vi "ReadByteArray.vi"(0 "Siemens Ctr":T1, 1 "# DB No.":u16, 2 "#items":u16, 3 "Item offset [byte]":u32, 4 "Address Areas":T2=132 items=["Input(I)"=129, "Output(Q)"=130, "Bit Memory(M)"=131, "Data(DB)"=132], 5 "error in (no error)":errorcluster, 6 "Bit/Byte":u8(ring)=2 items=["Boolen"=1, "Byte"=2]) -> (14 "Siemens Ctr out":T1, 15 "Byte Array":u8[](array[numeric]), 19 "error out":errorcluster)   [LabVIEW 2014, in "Simatic S7.lvlib"]
uses:
  Simatic S7.lvlib
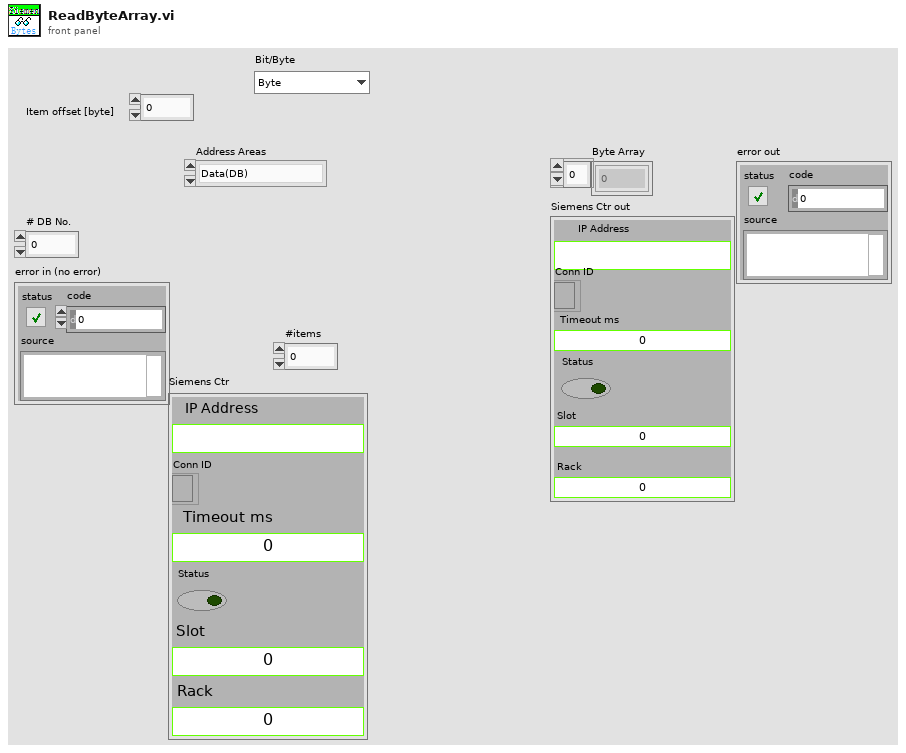
[diagram p1: front panel]
types:
  T1 = typedef "Simatic S7.lvlib/Siemens Ref.ctl" = cluster{"IP Address ":string, "Conn ID":refnum<k5>, "Timeout ms":i32, "Status":bool, "Slot":u16, "Rack":u16}
  T2 = typedef "Simatic S7.lvlib/Address Areas.ctl" = u8
  T3 = typedef "Data Type.ctl" = enum8{"Bit", "Byte (U8)", "Signed Byte (I8)", "Word (U16)", "Signed Word (I16)", "Long (U32)", "Signed Long (I32)", "Real (SGL)", "String"}
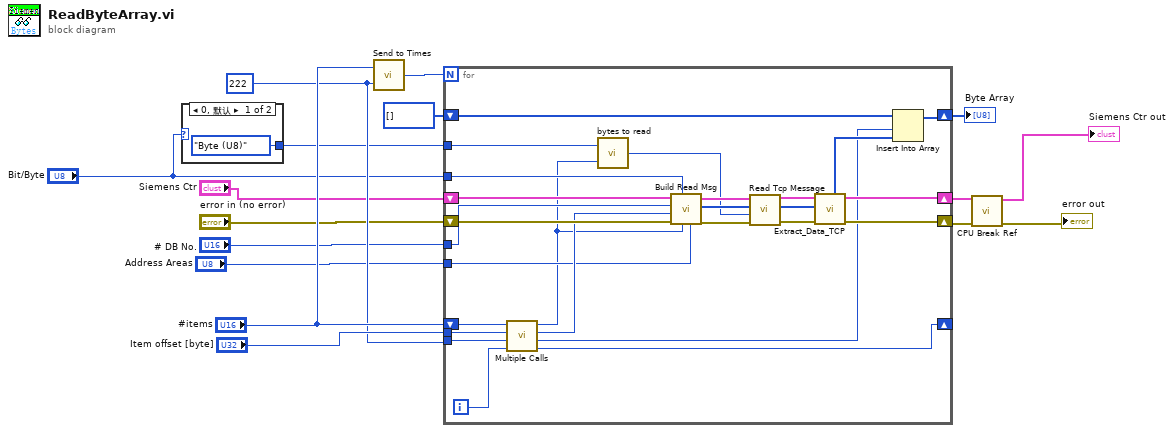
[diagram p0: block diagram]
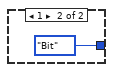
[diagram p2: hidden frame]
diagram:
  w13 = u8 222 ("max items per request")
  n1 = case shown="0, 默认" "Bit/Byte" {
    tunnel: [Data_Type."Byte (U8)" ("Data Type") Data_Type."Bit" ("Data Type")] -> w6
    frame 0, Default {
    }
    frame 1 {
    }
  }
  n2 = call "Send to Times.vi"("max items per request"=w13, "#items"="#items") -> ("for loop request"=w16:u16)
  n3 = for {
    N: w16 -> [_]
    tunnel: w6 -> [w44]
    tunnel: "Item offset [byte]" -> [w42]
    tunnel: w13 -> [w41]
    shift-right: [w40] -> _
    shift-left: "#items" -> [w43]
    tunnel: "Bit/Byte" -> [w36]
    tunnel: "# DB No." -> [w35]
    tunnel: "Address Areas" -> [w33]
    shift-right: [w26] -> w4
    shift-left: "error in (no error)" -> [w38]
    shift-right: [w23] -> w2
    shift-left: "Siemens Ctr" -> [w37]
    shift-right: [w21] -> w8
    shift-left: u8[] [] -> [w20]
    i -> [w39]
    n4 = call "Multiple Calls.vi"("For loop index"=w39, "Maximum Items per Request"=w41, "Item offset [byte]"=w42, "items #"=w43) -> ("Items left (shift register)"=w40:u16, "Result Array offset"=w19:i32, "Item Offset"=w34:u32, "Items to read"=w32:u16)  [unwired: 4 in]
    n5 = call "bytes to read.vi"("Items"=w32, "Data Type"=w44) -> ("Bytes to read"=w28:i32)
    n6 = call "Build Read Msg.vi"("Address Areas"=w33, "#items"=w32, "Bit/Byte"=w36, "error in (no error)"=w38, "#offset"=w34, "# DB No."=w35, "Siemens Ctr"=w37) -> ("error out"=w31:errorcluster, "Array Msg"=w29:u8[], "Siemens Ctr out"=w30:T1)  [unwired: 2 in]
    n7 = call "Read Tcp Message.vi"("error in (no error)"=w31, "bytes to read"=w28, "Request Message"=w29, "Siemens Ctr"=w30) -> ("error out"=w27:errorcluster, "Recieve Message"=w24:u8[], "S7 Connection out"=w25:T1)  [unwired: 4 in, 1 out]
    n8 = call "Extract_Data_TCP.vi"("error in (no error)"=w27, "Data Recieved"=w24, "Siemens Ctr in"=w25) -> ("error out"=w26:errorcluster, "Siemens Ctr"=w23:T1, "Data"=w22:u8[])  [unwired: 2 in, 4 out]
    n9 = Insert Into Array(array=w20, index=w19, new element=w22) -> (w21:u8[])
  }
  "Byte Array" <- w8
  n10 = call "CPU Break Ref.vi"("error in (no error)"=w4, "Siemens Ctr"=w2) -> ("error out"=→"error out":errorcluster, "Siemens Ctr out"=→"Siemens Ctr out":T1)  [unwired: 8 in]
